vi "Parse TC Setup.vi"(3 "INI File":string[](array[string])) -> (1 "TC Parameters":T1)   [LabVIEW 2015, in "Config Data.lvlib" / "Config Data_Text.lvclass"]
uses:
  Config Data_Text.lvclass
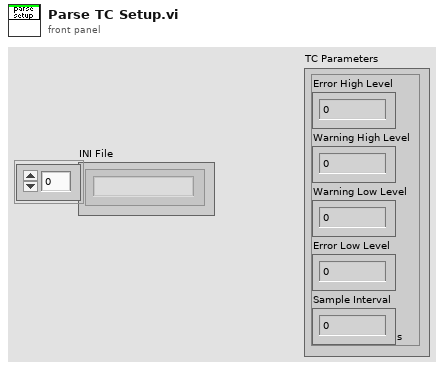
[diagram p1: front panel]
types:
  T1 = cluster{"Error High Level":dbl, "Warning High Level":dbl, "Warning Low Level":dbl, "Error Low Level":dbl, "Sample Interval":dbl[unit]}
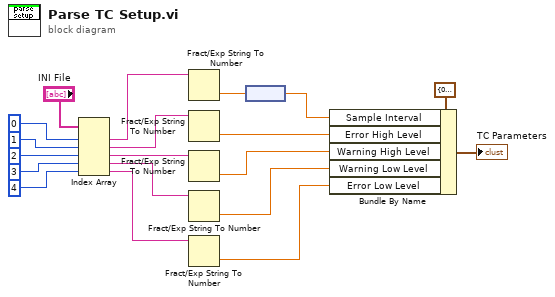
[diagram p0: block diagram]
diagram:
  n1 = Index Array(array="INI File", index #1=0 ("disabled index (col)"), index #2=1 ("disabled index (col)"), index #3=2 ("disabled index (col)"), index #4=3 ("disabled index (col)"), index #5=4 ("disabled index (col)")) -> (element #1=w11:string, element #2=w10:string, element #3=w9:string, element #4=w8:string, element #5=w7:string)
  n2 = Fract/Exp String To Number(string=w11) -> (number=w13:dbl)  [unwired: 3 in, 1 out]
  n3 = Fract/Exp String To Number(string=w10) -> (number=w15:dbl)  [unwired: 3 in, 1 out]
  n4 = Fract/Exp String To Number(string=w9) -> (number=w16:dbl)  [unwired: 3 in, 1 out]
  n5 = Fract/Exp String To Number(string=w8) -> (number=w17:dbl)  [unwired: 3 in, 1 out]
  n6 = Fract/Exp String To Number(string=w7) -> (number=w18:dbl)  [unwired: 3 in, 1 out]
  n7 = node(w13) -> (w14:dbl[unit])
  n8 = Bundle By Name(cluster=T1 {"Error High Level"=0.0, "Warning High Level"=0.0, "Warning Low Level"=0.0, "Error Low Level"=0.0, "Sample Interval"=0.0} ("TC Parameters"), "Sample Interval"=w14, "Error High Level"=w15, "Warning High Level"=w16, "Warning Low Level"=w17, "Error Low Level"=w18) -> (→"TC Parameters":T1)
